vi "Run.vi"(8 "error in (no error)":errorcluster, 9 "s on last turn":dbl, 10 "Maze (0: Empty, -1: Enemy. >0: Teammate":i32[][](array[numeric]), 11 "Class":refnum<class "Hesitant Wolf.lvclass">) -> (0 "error out":errorcluster, 1 "Direction":T1, 2 "Action":T2, 3 "Class":refnum<class "Hesitant Wolf.lvclass">, 4 "Replicated":refnum<class "Square.lvclass">)   [LabVIEW 2015, in "Hesitant Wolf.lvclass"]
uses:
  Hesitant Wolf.lvclass
  Type Defs/Action Enum.ctl
  Type Defs/Direction Enum.ctl
  Square/Square.lvclass
  Hesitant Wolf.lvclass/Hesitant Wolf.ctl
  SubVIs/Read-Only Globals.vi
  Type Defs/SB Type Defs.lvlib
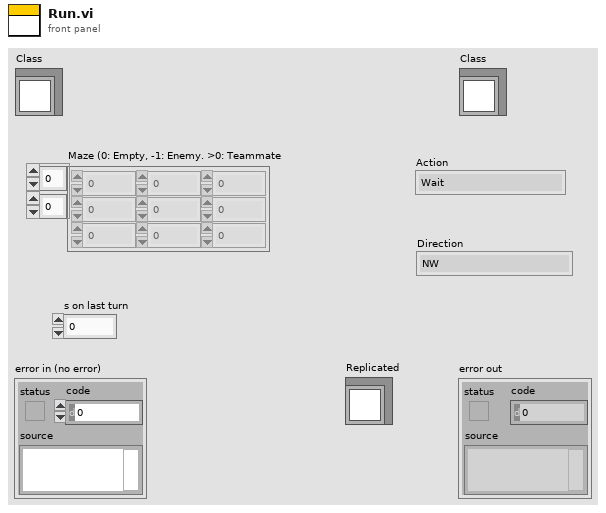
[diagram p1: front panel]
types:
  T1 = typedef "SB Type Defs.lvlib/Direction Enum.ctl" = enum16{"NW", "N", "NE", "E", "SE", "S", "SW", "W"}
  T2 = typedef "SB Type Defs.lvlib/Action Enum.ctl" = enum16{"Wait", "Move", "Attack", "Replicate"}
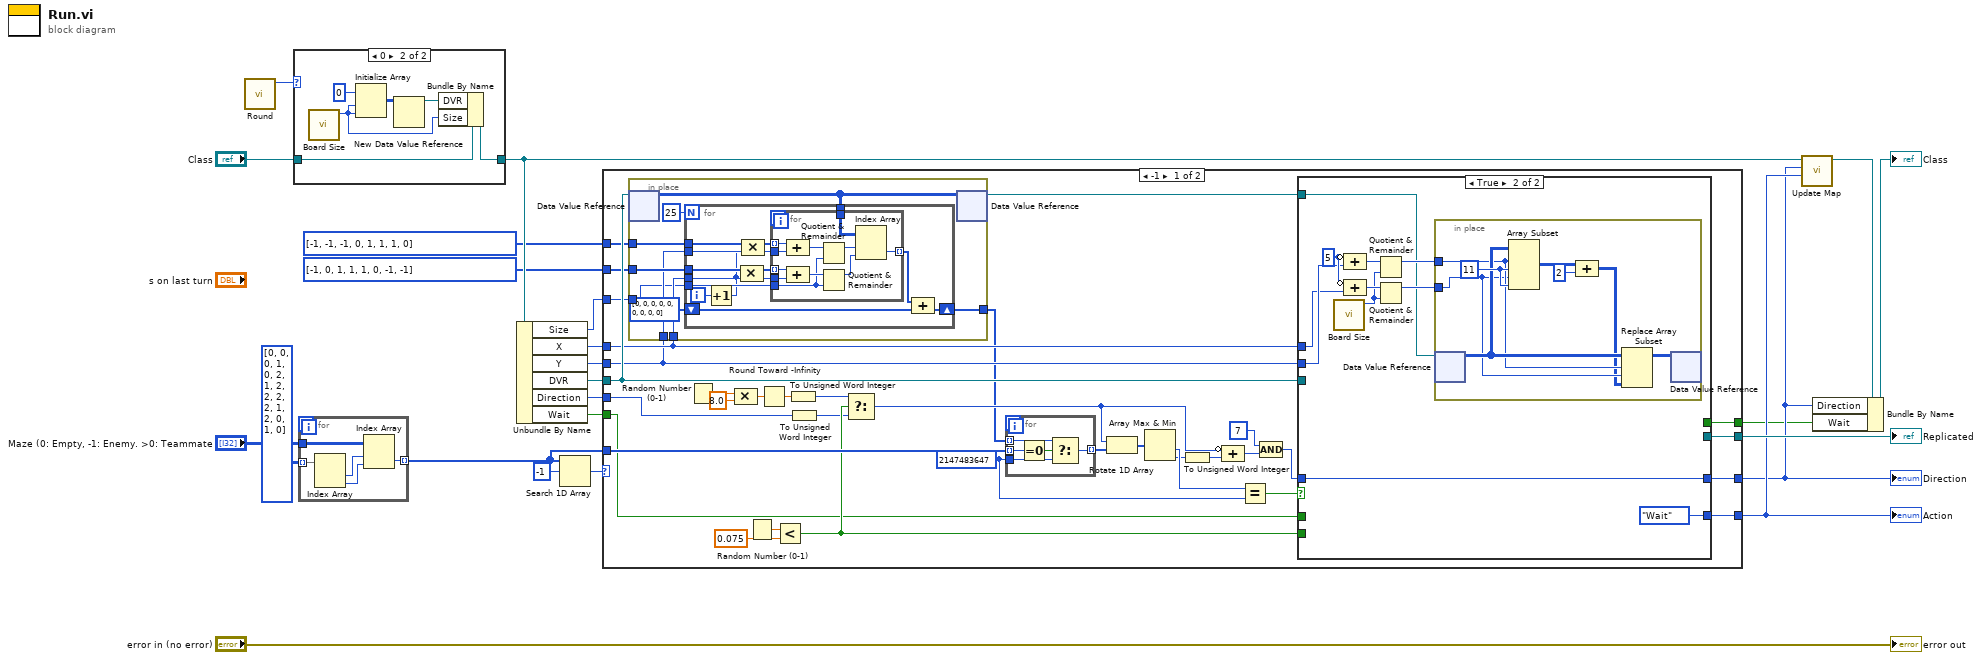
[diagram p0: block diagram]
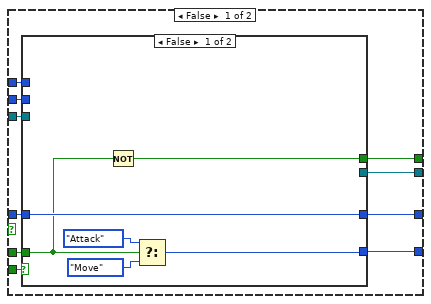
[diagram p3: hidden frame]
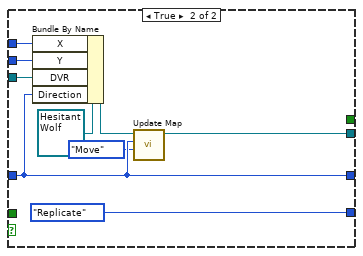
[diagram p4: hidden frame]
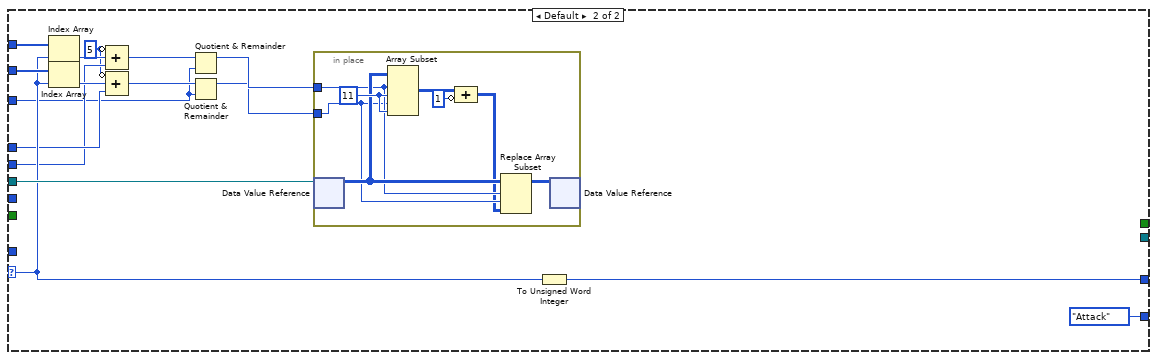
[diagram p5: hidden frame]
diagram:
  n1 = call "Round.vi"() -> ("Round"=w16:i32)  [unwired: 11 in]
  n2 = case shown="0" w16 {
    tunnel: "Class" -> [w24 w28]
    tunnel: [w24 w26] -> w11
    frame Default {
    }
    frame 0 {
      n3 = call "Board Size.vi"() -> ("Board Size"=w25:i32)  [unwired: 11 in]
      n4 = Initialize Array(0, w25, w25) -> (w29:i32[][])
      n5 = New Data Value Reference(data value=w29) -> (data value reference=w27:refnum<data-value>)  [unwired: 1 in, 1 out]
      n6 = Bundle By Name(cluster=w28, "DVR"=w27, "Size"=w25) -> (w26:refnum<class "Hesitant Wolf.lvclass">)
    }
  }
  n7 = for {
    tunnel: "Maze (0: Empty, -1: Enemy. >0: Teammate" -> [w35]
    tunnel: i32[][] [[0, 0], [0, 1], [0, 2], [1, 2], [2, 2], [2, 1], [2, 0], [1, 0]] -> [w34] mode=indexing
    tunnel: [w31] -> w18 mode=indexing
    n8 = Index Array(array=w34) -> (element #1=w33:i32, element #2=w32:i32)  [unwired: 2 in]
    n9 = Index Array(array=w35, index (row)=w33, index (col)=w32) -> (element=w31:i32)
  }
  n10 = Unbundle By Name(w11) -> ("Size"=w9:i32, "X"=w13:i32, "Y"=w12:i32, "DVR"=w14:refnum<data-value>, "Direction"=w3:T1, "Wait"=w2:bool)
  n11 = Search 1D Array(1D array=w18, element=-1) -> (index of element=w19:i32)  [unwired: 1 in]
  n12 = case shown="-1" w19 {
    selector: w19 -> [_ w164]
    tunnel: [w69 w153] -> w5
    tunnel: [w70 Action_Enum."Attack" ("Action")] -> w10
    tunnel: w18 -> [w65 _]
    tunnel: [w68 _] -> w17
    tunnel: w14 -> [w64 w167]
    tunnel: w13 -> [w50 w162]
    tunnel: w12 -> [w49 w158]
    tunnel: i32[] [-1, -1, -1, 0, 1, 1, 1, 0] -> [w63 w166]
    tunnel: i32[] [-1, 0, 1, 1, 1, 0, -1, -1] -> [w62 w165]
    tunnel: w9 -> [w61 w157]
    tunnel: w3 -> [w46 _]
    tunnel: w2 -> [w37 _]
    tunnel: [w36 _] -> w1
    frame -1 {
      w60 = 2147483647
      n13 = in-place {
        in-place-border: w63 -> [w78]
        in-place-border: w62 -> [w77]
        in-place-border: w49 -> [w76]
        in-place-border: w50 -> [w75]
        in-place-border: w61 -> [w74]
        in-place-border: [w72] -> w38
        n14 = in-place-dvr #1(w64) -> (w79:i32[][])  [unwired: 1 out]
        n15 = for {
          N: 25 -> [_]
          tunnel: w79 -> [w92]
          tunnel: w78 -> [w91]
          tunnel: w77 -> [w90]
          tunnel: w76 -> [w89]
          tunnel: w75 -> [w88]
          tunnel: w74 -> [w87]
          shift-right: [w81] -> w72
          shift-left: i32[] [0, 0, 0, 0, 0, 0, 0, 0, 0] -> [w80]
          i -> [w86]
          n16 = Increment(x=w86) -> (x+1=w83:i32)
          n17 = Compound Arithmetic op=MULTIPLY(w90, w83) -> (w85:i32[])
          n18 = Compound Arithmetic op=MULTIPLY(w91, w83) -> (w84:i32[])
          n19 = for {
            tunnel: w92 -> [w103]
            tunnel: w84 -> [w99] mode=indexing
            tunnel: w85 -> [w98] mode=indexing
            tunnel: w89 -> [w97]
            tunnel: w88 -> [w96]
            tunnel: w87 -> [w95]
            tunnel: [w93] -> w82 mode=indexing
            n20 = Compound Arithmetic op=ADD(w99, w97) -> (w102:i32)
            n21 = Compound Arithmetic op=ADD(w98, w96) -> (w101:i32)
            n22 = Quotient & Remainder(x=w102, y=w95) -> (x-y*floor(x/y)=w100:i32)  [unwired: 1 out]
            n23 = Quotient & Remainder(x=w101, y=w95) -> (x-y*floor(x/y)=w94:i32)  [unwired: 1 out]
            n24 = Index Array(array=w103, index (row)=w100, index (col)=w94) -> (element=w93:i32)
          }
          n25 = Compound Arithmetic op=ADD(w82, w80) -> (w81:i32[])
        }
        n26 = in-place-dvr #1(w79) -> (w39:refnum<data-value>)  [unwired: 1 out]
      }
      n27 = Random Number (0-1)() -> (number: 0 to 1=w53:dbl)
      n28 = Compound Arithmetic op=MULTIPLY(w53, 8.0 ("value")) -> (w55:dbl)
      n29 = Random Number (0-1)() -> (number: 0 to 1=w66:dbl)
      n30 = Round Toward -Infinity(1:w55) -> (0:w56:dbl)
      n31 = Less?(x=w66, y=0.075) -> (x < y?=w47:bool)
      n32 = To Unsigned Word Integer(number=w56) -> (unsigned 16bit integer=w48:u16)
      n33 = To Unsigned Word Integer(number=w46) -> (unsigned 16bit integer=w44:u16)
      n34 = Select(t=w48, s=w47, f=w44) -> (s? t:f=w45:u16)
      n35 = for {
        tunnel: w65 -> [w152] mode=indexing
        tunnel: w38 -> [w150] mode=indexing
        tunnel: w60 -> [w149]
        tunnel: [w148] -> w58 mode=indexing
        n36 = Equal To 0?(x=w152) -> (x = 0?=w151:bool)
        n37 = Select(t=w150, s=w151, f=w149) -> (s? t:f=w148:i32)
      }
      n38 = Rotate 1D Array(1:w58, 2:w45) -> (0:w57:i32[])
      n39 = Array Max & Min(array=w57) -> (min value=w52:i32, min index (indices)=w51:i32)  [unwired: 2 out]
      n40 = To Unsigned Word Integer(number=w51) -> (unsigned 16bit integer=w43:u16)
      n41 = Compound Arithmetic op=ADD(invert w45, w43) -> (w42:u16)
      n42 = Equal?(x=w52, y=w60) -> (x = y?=w59:bool)
      n43 = Compound Arithmetic op=AND(u16 7 ("value"), w42) -> (w41:u16)
      n44 = case shown="True" w59 {
        tunnel: [w113 Action_Enum."Wait" ("y")] -> w70
        tunnel: [w112 w138] -> w69
        tunnel: [w111 _] -> w68
        tunnel: w47 -> [w110 _]
        tunnel: w41 -> [w109 w138]
        tunnel: w64 -> [w108 _]
        tunnel: w50 -> [w107 w130]
        tunnel: w49 -> [w106 w131]
        tunnel: w39 -> [_ w132]
        tunnel: w37 -> [w105 _]
        tunnel: [w104 _] -> w36
        frame False {
          n45 = case shown="False" w110 {
            tunnel: [w116 Action_Enum."Replicate" ("y")] -> w113
            tunnel: [w119 w123] -> w112
            tunnel: [_ w124] -> w111
            tunnel: w109 -> [w119 w123]
            tunnel: w108 -> [_ w126]
            tunnel: w107 -> [_ w121]
            tunnel: w106 -> [_ w120]
            tunnel: w105 -> [w115 _]
            tunnel: [w114 _] -> w104
            frame False {
              n46 = Not(x=w115) -> (.not. x?=w114:bool)
              n47 = Select(t=Action_Enum."Attack" ("y"), s=w115, f=Action_Enum."Move" ("y")) -> (s? t:f=w116:T2)
            }
            frame True {
              n48 = Bundle By Name(cluster=refnum<class "Hesitant Wolf.lvclass"> refnum ("Lone Wolf.lvclass"), "X"=w121, "Y"=w120, "DVR"=w126, "Direction"=w123) -> (w125:refnum<class "Hesitant Wolf.lvclass">)
              n49 = call "Update Map.vi"("Action"=Action_Enum."Move", "Direction"=w123, "Class"=w125) -> ("Class"=w124:refnum<class "Hesitant Wolf.lvclass">)  [unwired: 8 in]
            }
          }
        }
        frame True {
          w135 = 5 ("value")
          n50 = call "Board Size.vi"() -> ("Board Size"=w129:i32)  [unwired: 11 in]
          n51 = Compound Arithmetic op=ADD(invert w135, w131) -> (w136:i32)
          n52 = Compound Arithmetic op=ADD(invert w135, w130) -> (w137:i32)
          n53 = Quotient & Remainder(x=w136, y=w129) -> (x-y*floor(x/y)=w134:i32)  [unwired: 1 out]
          n54 = Quotient & Remainder(x=w137, y=w129) -> (x-y*floor(x/y)=w133:i32)  [unwired: 1 out]
          n55 = in-place {
            in-place-border: w134 -> [w142]
            in-place-border: w133 -> [w141]
            w147 = 11 ("length")
            n56 = in-place-dvr #2(w132) -> (w144:i32[][])  [unwired: 1 out]
            n57 = Array Subset(array=w144, index (row)=w142, length (row)=w147, index (col)=w141, length (col)=w147) -> (w146:i32[][])
            n58 = Compound Arithmetic op=ADD(w146, 2 ("length")) -> (w140:i32[][])
            n59 = Replace Array Subset(array=w144, new element=w140, index (row)=w142, index (col)=w141) -> (w143:i32[][])
            n60 = in-place-dvr #2(w143) -> ()  [unwired: 2 out]
          }
        }
      }
    }
    frame Default {
      w156 = 5 ("value")
      n61 = Index Array(array=w166, index=w164) -> (element=w159:i32)
      n62 = Index Array(array=w165, index=w164) -> (element=w163:i32)
      n63 = Compound Arithmetic op=ADD(invert w156, w159, w158) -> (w160:i32)
      n64 = Compound Arithmetic op=ADD(invert w156, w163, w162) -> (w161:i32)
      n65 = Quotient & Remainder(x=w160, y=w157) -> (x-y*floor(x/y)=w155:i32)  [unwired: 1 out]
      n66 = Quotient & Remainder(x=w161, y=w157) -> (x-y*floor(x/y)=w154:i32)  [unwired: 1 out]
      n67 = in-place {
        in-place-border: w155 -> [w171]
        in-place-border: w154 -> [w170]
        w176 = 11 ("length")
        n68 = in-place-dvr #3(w167) -> (w173:i32[][])  [unwired: 1 out]
        n69 = Array Subset(array=w173, index (row)=w171, length (row)=w176, index (col)=w170, length (col)=w176) -> (w175:i32[][])
        n70 = Compound Arithmetic op=ADD(w175, invert 1 ("length")) -> (w169:i32[][])
        n71 = Replace Array Subset(array=w173, new element=w169, index (row)=w171, index (col)=w170) -> (w172:i32[][])
        n72 = in-place-dvr #3(w172) -> ()  [unwired: 2 out]
      }
      n73 = To Unsigned Word Integer(number=w164) -> (unsigned 16bit integer=w153:u16)
    }
  }
  "Action" <- w10
  "Direction" <- w5
  "Replicated" <- w17
  n74 = call "Update Map.vi"("Action"=w10, "Direction"=w5, "Class"=w11) -> ("Class"=w6:refnum<class "Hesitant Wolf.lvclass">)  [unwired: 8 in]
  n75 = Bundle By Name(cluster=w6, "Direction"=w5, "Wait"=w1) -> (→"Class":refnum<class "Hesitant Wolf.lvclass">)
  "error out" <- "error in (no error)"
